vi "GUI_HPDMAP.vi"() -> ()   [LabVIEW 2013]
uses:
  Shared/GUI_Template/GUI_master/tcp_new_data_event.ctl
  Shared/GUI_Template/GUI_master/tcp new data cluster.ctl
  <vilib>/vision/Image Controls.llb/IMAQ Image.ctl
panel:
  in  "GUIdevice 4":string="HPD_EnergyMeter"
  in  "data::4":dbl=25.5 caption="Energy Reading" min=0.0 max=300000000.0 format="%_4f"
  in  "GUIdevice 3":string="HPD Filterwheel"
  in  "pos.Channel0::3":enum16{"1", "2", "3", "4", "5", "6"}(ring) caption="Filter Position"
  out "temporalFWHM::2":dbl caption="Pulse Width" min=0.0 max=50000.0
  in  "triggermode::2":T1(ring) caption="Trigger Mode"
  in  "exposure::2":dbl=0.001 caption="Exposure" min=0.0453 max=10000.0 format="%_4p"
  in  "cameraselect::2":enum16{"temporal CAM", "spatial CAM"}(ring) caption="Select Camera"
  out "SpatialImage::2":T2(plugin-control) caption="Spatial Image"
  out "retrievedFrogTrace::2":T2(plugin-control) caption="Retrieved Frog Trace"
  out "frogTrace::2":T2(plugin-control) caption="FROG Trace"
  in  "GUIdevice 2":string="Frog_HPD"
  in  "position::1":dbl caption="Position" min=0.0 max=395.0 format="%#_6p"
  in  "GUIdevice 1":string="HPDTelescopeStage"
  in  "stop":bool
  out "error IO 2":errorcluster
  out "tcp data event":T3
  in  "HPDTEL":u16(ring)
  # "HPD Area MAP"
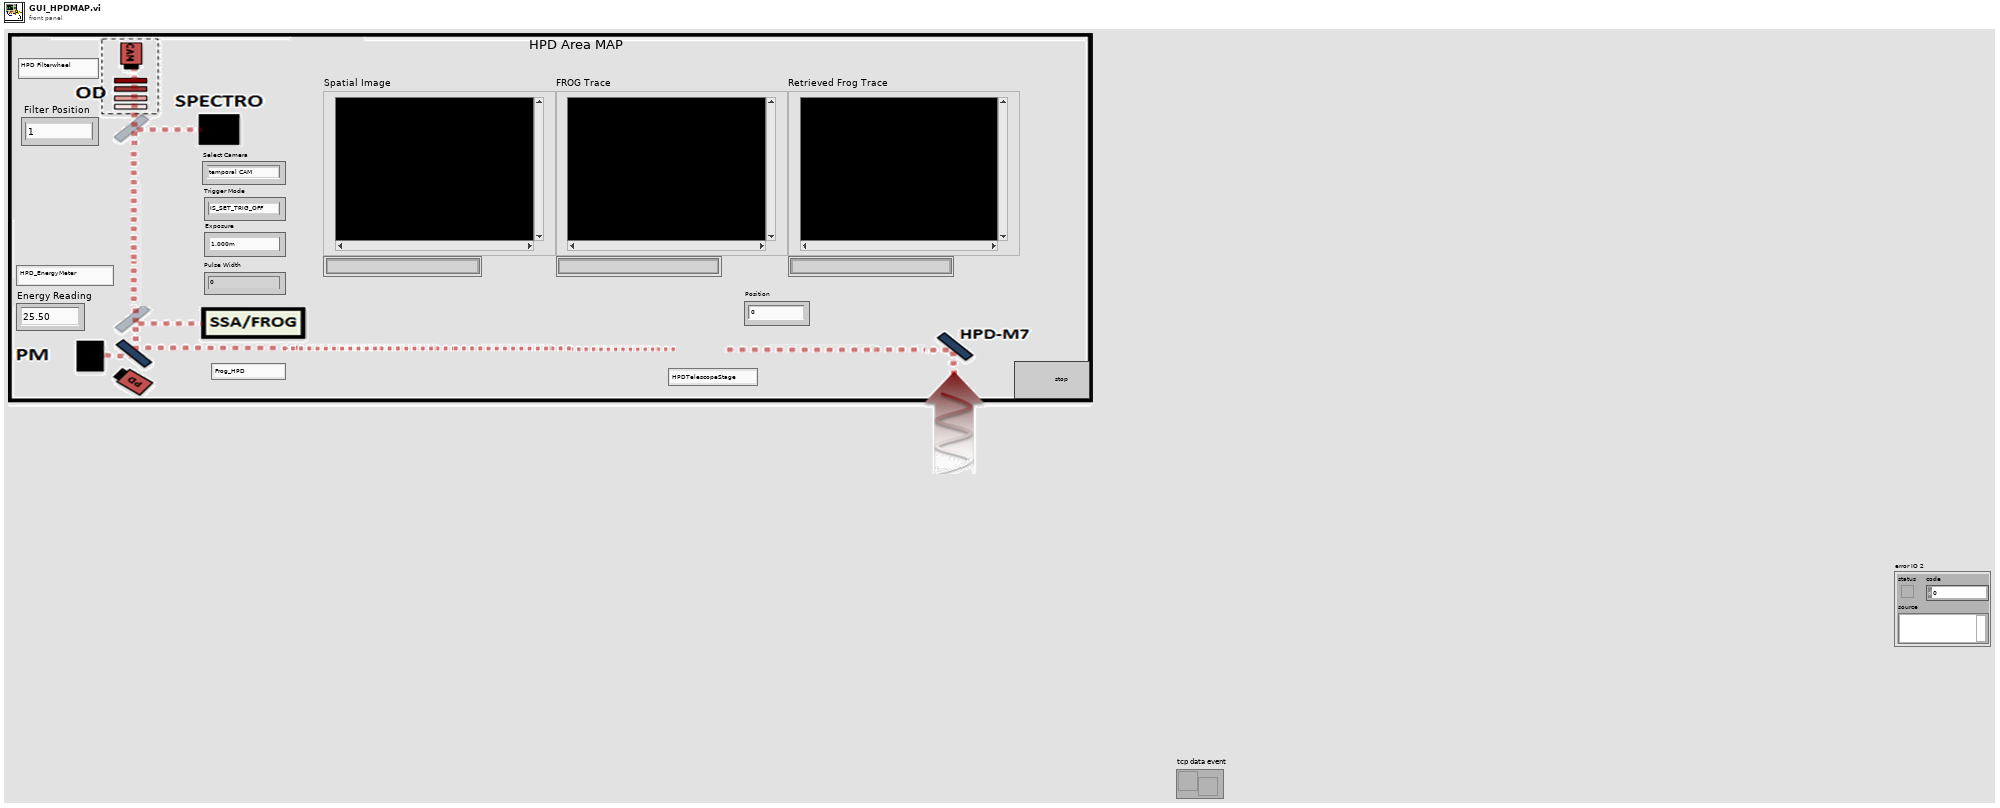
[diagram p1: front panel]
types:
  T1 = enum16{"IS_SET_TRIG_OFF", "IS_SET_TRIG_HI_LO", "IS_SET_TRIG_LO_HI", "IS_SET_TRIG_SOFTWARE", "IS_GET_EXTERNAL_TRIGGER", "IS_GET_TRIGGER_STATUS"}
  T2 = typedef "IMAQ Image.ctl" = refnum<image>
  T3 = typedef "tcp_new_data_event.ctl" = refnum<user-event>
  T4 = typedef "tcp new data cluster.ctl" = cluster{"EventEnum":enum16{"new data", "connection status update"}, "Device name":string}
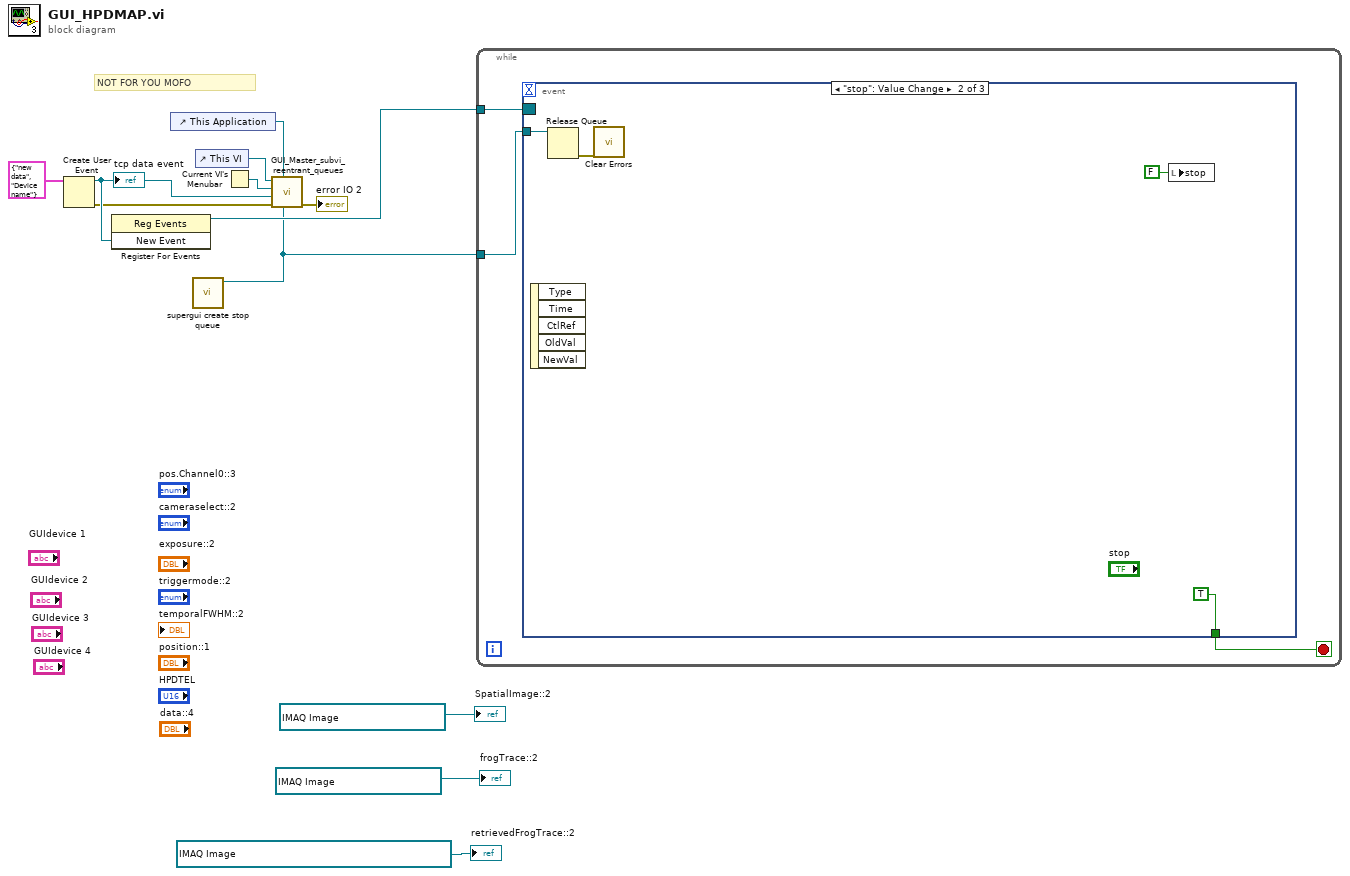
[diagram p0: block diagram]
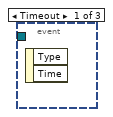
[diagram p2: hidden frame]
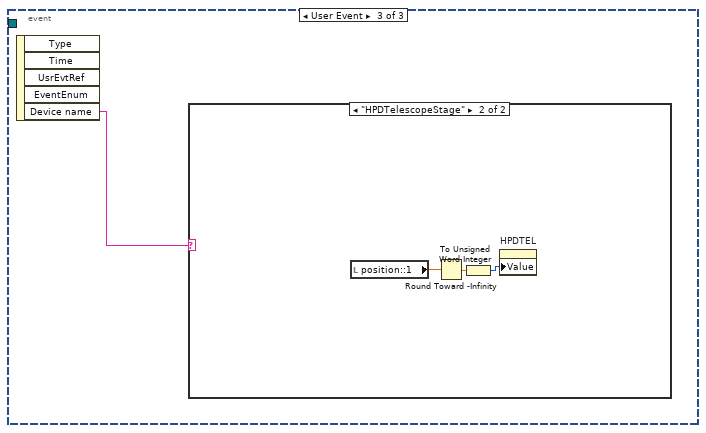
[diagram p3: hidden frame]
diagram:
  # "NOT FOR YOU MOFO"
  n1 = Create User Event(user event datatype=T4 {"EventEnum"=enum."new data", "Device name"="Device name"} ("New Event")) -> (user event=w11:refnum<user-event>, error out=w10:errorcluster)  [unwired: 1 in]
  "tcp data event" <- w11
  n2 = register-events(w11) -> (reference out=w5:refnum<event-registration>)  [unwired: 2 in, 1 out]
  n3 = control-ref of="This Application"() -> (w12:refnum<vi>)
  n4 = call "supergui create stop queue.vi"() -> ("STOP Queue out"=w1:refnum<queue>)  [unwired: 11 in]
  n5 = control-ref of="This VI"() -> (w7:refnum<vi>)
  n6 = Current VI's Menubar() -> (w8:refnum<k9>)
  n7 = call "GUI_Master_subvi_reentrant_queues.vi"("STOP Queue in"=w1, "This Application"=w12, "error in (no error)"=w10, "tcp data event"=w11, "Caller menu reference"=w8, "Caller VI ref"=w7) -> ("error out"=→"error IO 2":errorcluster)  [unwired: 5 in]
  n8 = while {
    tunnel: w5 -> [w14]
    tunnel: w1 -> [w13]
    stop <- w15 stop-if-true
    n9 = event shown="[1] \"stop\": Value Change" {
      selector: w14 -> [_ _ _]
      dyn-events: _ -> [_ _ _]
      timeout: _ -> [_ _ _]
      tunnel: [_ TRUE _] -> w15
      tunnel: w13 -> [_ w17 _]
      event Timeout {
        n10 = event-data() -> ()  [unwired: 1 in, 2 out]
      }
      event "stop": Value Change {
        n11 = event-data() -> ()  [unwired: 1 in, 5 out]
        n12 = Release Queue(queue=w17) -> (error out=w16:errorcluster)  [unwired: 2 in, 2 out]
        n13 = call <vilib>:"Clear Errors.vi"("error in (no error)"=w16) -> ()  [unwired: 6 in, 1 out]
        n14 = local write "stop"(FALSE ("stop")) -> ()
      }
      event User Event {
        n15 = event-data() -> ("Device name"=w20:string)  [unwired: 1 in, 4 out]
        n16 = case shown="\"HPDTelescopeStage\"" w20 {
          frame "False", Default {
          }
          frame "HPDTelescopeStage" {
            n17 = local read "position::1"() -> (w22:dbl)
            n18 = Round Toward -Infinity(1:w22) -> (0:w23:dbl)
            n19 = To Unsigned Word Integer(number=w23) -> (unsigned 16bit integer=w21:u16)
            n20 = property on="HPDTEL" class="Ring (strict)"("Value"=w21) -> ()  [unwired: 2 in, 2 out]
          }
        }
      }
    }
  }
  "frogTrace::2" <- T2 refnum ("New Image")
  "retrievedFrogTrace::2" <- T2 refnum ("New Image")
  "SpatialImage::2" <- T2 refnum ("New Image")
